vi "Do Comparison.vi"(8 "error in (no error)":errorcluster, 10 "Compare Timestamp":timestamp, 11 "Time Filters in":refnum<class "Time Filters.lvclass">) -> (0 "error out":errorcluster, 2 "Filtered":bool)   [LabVIEW 2016, in "Assert API Components.lvlib" / "Time Filters.lvclass"]
uses:
  Time Filters.lvclass
  Time Filters.lvclass/Time Filters.ctl
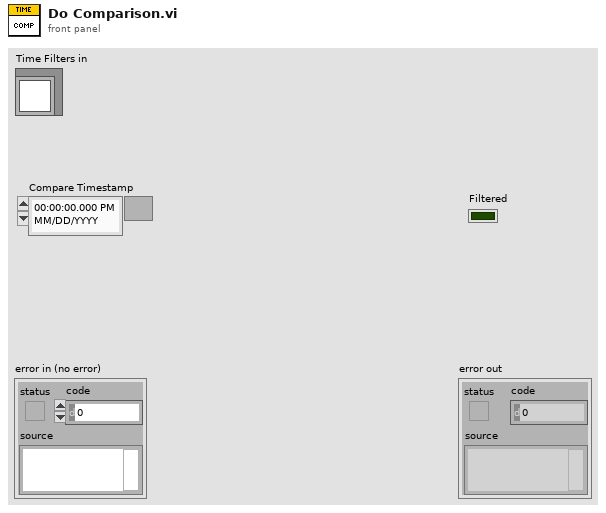
[diagram p1: front panel]
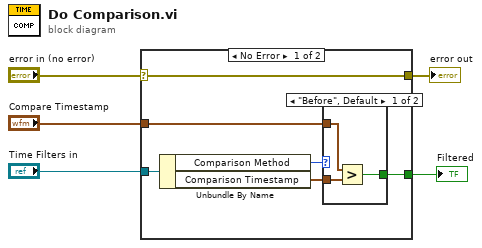
[diagram p0: block diagram]
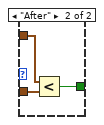
[diagram p2: hidden frame]
diagram:
  n1 = case shown="No Error" "error in (no error)" {
    selector: "error in (no error)" -> [w11 w18]
    tunnel: [w11 w18] -> w4
    tunnel: "Time Filters in" -> [w10 _]
    tunnel: "Compare Timestamp" -> [w7 _]
    tunnel: [w6 _] -> w1
    frame No Error {
      n2 = Unbundle By Name(w10) -> ("Comparison Method"=w9:enum16{"Before", "After"}, "Comparison Timestamp"=w8:timestamp)
      n3 = case shown="\"Before\", Default" w9 {
        tunnel: w8 -> [w13 w16]
        tunnel: w7 -> [w14 w17]
        tunnel: [w12 w15] -> w6
        frame "Before", Default {
          n4 = Greater?(x=w14, y=w13) -> (0:w12:bool)
        }
        frame "After" {
          n5 = Less?(x=w17, y=w16) -> (x < y?=w15:bool)
        }
      }
    }
    frame Error {
    }
  }
  "error out" <- w4
  "Filtered" <- w1
